vi "init.vi"(8 "error in":errorcluster, 10 "module configuration":refnum<class "TBM module configuration.lvclass">, 11 "module in":refnum<class "E2E Runtime (UDP).lvclass">) -> (0 "error out":errorcluster, 1 "data allocations":T1, 2 "execution settings":T4, 3 "module out":refnum<class "E2E Runtime (UDP).lvclass">)   [LabVIEW 2015, in "E2E Runtime (UDP).lvclass"]
doc: "Provides an interface for initializing a module at runtime. While this interface performs no operations, a child should provide an override which may open any necessary references or sessions, allocate necessary memory, and perform any final configuration validataion before providing the full configuration <b>execution data</b> to the calling process."
uses:
  E2E Runtime (UDP).lvclass
  <vilib>/NI/Tag Bus Module Framework/module configuration/TBM module configuration.lvclass
  <vilib>/NI/Tag Bus Module Framework/runtime/execution settings.ctl
  <vilib>/NI/Tag Bus Module Framework/channel/data tables.ctl
  <vilib>/NI/Tag Bus/dictionary/data dictionary.lvclass
  <vilib>/NI/Tag Bus/dictionary table pair.ctl
  <vilib>/NI/Tag Bus/table/data table.ctl
  configuration/E2E Tag Exchange configuration.lvclass
  <vilib>/NI/Configuration Framework/serializable configuration/NISE_CEF_serializable configuration.lvclass/NISE_CEF_serializable configuration.ctl
  configuration/E2E Tag Exchange configuration.lvclass/E2E Tag Exchange configuration.ctl
  E2E Runtime (UDP).lvclass/E2E Runtime (UDP).ctl
  <vilib>/Utility/LVClass/Get LV Class Name.vi
  <vilib>/NI/Configuration Framework/error generator/NISE_error generator.vi
  <vilib>/NI/Tag Bus Module Framework/channel/TBM channel.lvclass
  <vilib>/NI/Tag Bus Module Framework/runtime/TBM module execution interface.lvclass
  <vilib>/NI/Configuration Framework/serializable configuration/NISE_CEF_serializable configuration.lvclass
  <vilib>/NI/Tag Bus/tag bus.lvlib
  <vilib>/NI/Tag Bus/table/data table.lvlib
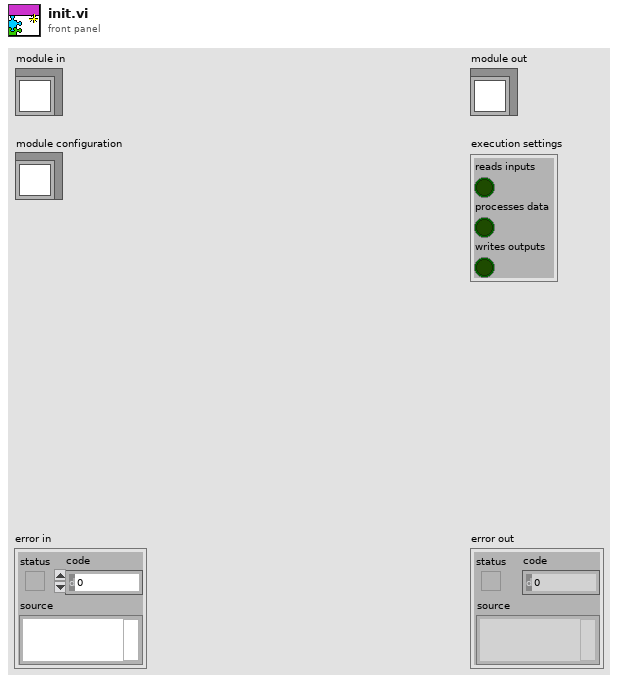
[diagram p1: front panel]
types:
  T1 = typedef "TBM channel.lvclass/data tables.ctl" = cluster{"input data":T2, "processing parameter":T2, "processing result":T2, "output data":T2}
  T2 = typedef "tag bus.lvlib/dictionary table pair.ctl" = cluster{"data dictionary":refnum<class "data dictionary.lvclass">, "data table":T3}
  T3 = typedef "tag bus.lvlib/data table.lvlib/data table.ctl" = cluster{"Double":dbl[], "Single":sgl[], "I64":i64[], "I32":i32[], "I16":i16[], "I8":i8[], "U64":u64[], "U32":u32[], "U16":u16[], "U8":u8[], "Boolean":bool[], "String":string[], "Array of Double":cluster{"DBL Array":dbl[]}[], "Array of Single":cluster{"SGL Array":sgl[]}[], "Array of I64":cluster{"I64 Array":i64[]}[], "Array of I32":cluster{"I32 Array":i32[]}[], "Array of I16":cluster{"I16 Array":i16[]}[], "Array of I8":cluster{"I8 Array":i8[]}[], "Array of U64":cluster{"U64 Array":u64[]}[], "Array of U32":cluster{"U32 Array":u32[]}[], "Array of U16":cluster{"U16 Array":u16[]}[], "Array of U8":cluster{"U8 Array":u8[]}[], "Array of Boolean":cluster{"Boolean Array":bool[]}[], "Array of String":cluster{"String Array":string[]}[]}
  T4 = typedef "TBM module execution interface.lvclass/execution settings.ctl" = cluster{"reads inputs":bool, "processes data":bool, "writes outputs":bool}
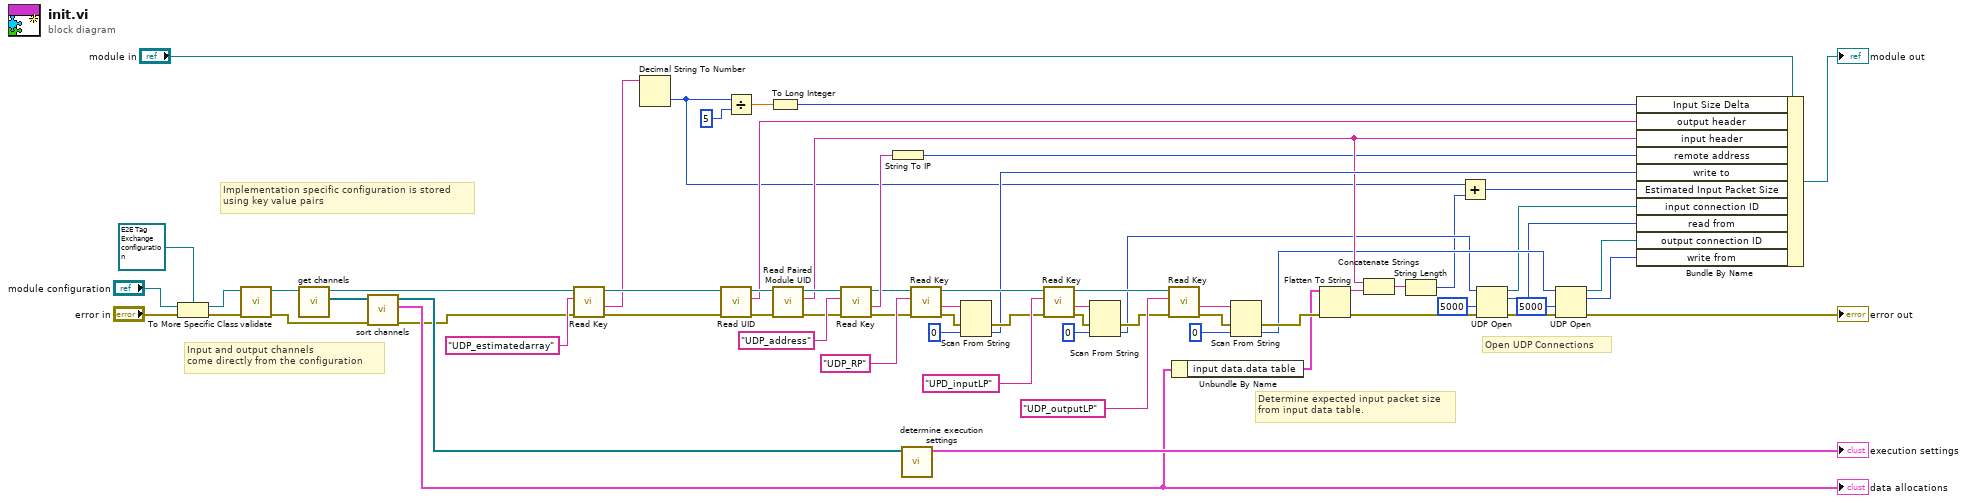
[diagram p0: block diagram]
diagram:
  # "Determine expected input packet size\nfrom input data table."
  # "Open UDP Connections"
  # "Input and output channels\ncome directly from the configuration"
  # "Implementation specific configuration is stored\nusing key value pairs"
  n1 = To More Specific Class(target class=refnum<class "E2E Tag Exchange configuration.lvclass"> refnum ("E2E configuration"), reference="module configuration", error in="error in") -> (specific class reference=w64:refnum<class "E2E Tag Exchange configuration.lvclass">, error out=w65:errorcluster)
  n2 = call-dynamic "validate.vi"("error in"=w65, "E2E Tag Exchange configuration in"=w64) -> ("error out"=w61:errorcluster, "E2E Tag Exchange configuration out"=w63:refnum<class "E2E Tag Exchange configuration.lvclass">)  [unwired: 8 in]
  n3 = call-dynamic "get channels.vi"("E2E configuration in"=w63) -> ("channels"=w62:refnum<class "TBM channel.lvclass">[], "E2E configuration out"=w6:refnum<class "E2E Tag Exchange configuration.lvclass">)  [unwired: 9 in]
  n4 = call <vilib>:"sort channels.vi"("error in"=w61, "channels in"=w62) -> ("error out"=w7:errorcluster, "data allocations"=w22:T1, "channels out"=w60:refnum<class "TBM channel.lvclass">[])  [unwired: 7 in]
  "data allocations" <- w22
  n5 = call "Read Key.vi"("error in"=w7, "Key"="UDP_estimatedarray", "E2E configuration in"=w6) -> ("error out"=w8:errorcluster, "Value"=w4:string, "E2E configuration out"=w9:refnum<class "E2E Tag Exchange configuration.lvclass">)  [unwired: 6 in]
  n6 = Decimal String To Number(string=w4) -> (number=w3:i32)  [unwired: 2 in, 1 out]
  n7 = call <vilib>:"Read UID.vi"("error in"=w8, "configuration in"=w9) -> ("error out"=w52:errorcluster, "instance id"=w46:string, "configuration out"=w53:refnum<class "E2E Tag Exchange configuration.lvclass">)  [unwired: 7 in]
  n8 = Divide(x=w3, y=5) -> (x/y=w10:dbl)
  n9 = To Long Integer(number=w10) -> (32bit integer=w5:i32)
  n10 = call "Read Paired Module UID.vi"("error in (no error)"=w52, "E2E Tag Exchange configuration in"=w53) -> ("error out"=w19:errorcluster, "Paired Module UID"=w25:string, "E2E Tag Exchange configuration out"=w45:refnum<class "E2E Tag Exchange configuration.lvclass">)  [unwired: 7 in]
  n11 = call "Read Key.vi"("error in"=w19, "Key"="UDP_address", "E2E configuration in"=w45) -> ("error out"=w42:errorcluster, "Value"=w44:string, "E2E configuration out"=w43:refnum<class "E2E Tag Exchange configuration.lvclass">)  [unwired: 6 in]
  n12 = String To IP(1:w44) -> (0:w20:u32)
  n13 = call <vilib>:"determine execution settings.vi"("channels"=w60) -> ("execution settings"=→"execution settings":T4)  [unwired: 10 in]
  n14 = call "Read Key.vi"("error in"=w42, "Key"="UDP_RP", "E2E configuration in"=w43) -> ("error out"=w41:errorcluster, "Value"=w29:string, "E2E configuration out"=w38:refnum<class "E2E Tag Exchange configuration.lvclass">)  [unwired: 6 in]
  n15 = Scan From String(input string=w29, error in=w41, default 1=u16 0 ("remote port")) -> (error out=w37:errorcluster, output 1=w35:u16)  [unwired: 2 in, 2 out]
  n16 = call "Read Key.vi"("error in"=w37, "Key"="UPD_inputLP", "E2E configuration in"=w38) -> ("error out"=w36:errorcluster, "Value"=w28:string, "E2E configuration out"=w33:refnum<class "E2E Tag Exchange configuration.lvclass">)  [unwired: 6 in]
  n17 = Scan From String(input string=w28, error in=w36, default 1=u16 0 ("remote port")) -> (error out=w32:errorcluster, output 1=w17:u16)  [unwired: 2 in, 2 out]
  n18 = call "Read Key.vi"("error in"=w32, "Key"="UDP_outputLP", "E2E configuration in"=w33) -> ("error out"=w27:errorcluster, "Value"=w30:string)  [unwired: 6 in, 1 out]
  n19 = Unbundle By Name(w22) -> ("input data.data table"=w21:T3)
  n20 = Scan From String(input string=w30, error in=w27, default 1=u16 0 ("remote port")) -> (error out=w26:errorcluster, output 1=w18:u16)  [unwired: 2 in, 2 out]
  n21 = Flatten To String(anything=w21, error in (no error)=w26) -> (data string=w47:string, error out=w24:errorcluster)  [unwired: 2 in, 1 out]
  n22 = Concatenate Strings(w25, w47) -> (w48:string)
  n23 = String Length(string=w48) -> (length=w1:i32)
  n24 = Add(x=w3, y=w1) -> (x+y=w2:i32)
  n25 = UDP Open(8:w24, 9:5000 ("timeout ms (25000)"), 11:w17) -> (port=w13:refnum<k16>, 0:w58:errorcluster, 2:w16:u16)  [unwired: 2 in]
  n26 = UDP Open(8:w58, 9:5000 ("timeout ms (25000)"), 11:w18) -> (port=w14:refnum<k16>, 0:→"error out":errorcluster, 2:w15:u16)  [unwired: 2 in]
  n27 = Bundle By Name(cluster="module in", "Input Size Delta"=w5, "output header"=w46, "input header"=w25, "remote address"=w20, "write to"=w35, "Estimated Input Packet Size"=w2, "input connection ID"=w13, "read from"=w16, "output connection ID"=w14, "write from"=w15) -> (→"module out":refnum<class "E2E Runtime (UDP).lvclass">)
